vi "Create Analog DataSet MultiRow DataQ.vi"(8 "error in (no error)":errorcluster, 9 "Select":T1, 10 "TaskName":string, 11 "DataQueues in":refnum<class "DataQueues.lvclass">) -> (0 "error out":errorcluster, 2 "TaskName out":string, 3 "DataQueues out":refnum<class "DataQueues.lvclass">)   [LabVIEW 2017, in "DataQueues.lvclass"]
doc: "Developed by Kevin Thompson\nkevin@thompsonengineering.net\n\nCopyright 2018-2020\nThompson Engineering, LLC"
uses:
  DataQueues.lvclass
  DataTypes/DataQ SelectType--enum.ctl
  DataTypes/Analog DataSet MultiRow--cluster.ctl
  DataTypes/DataQ Ref DictNode--cluster.ctl
  DataQueues.lvclass/DataQueues.ctl
  Accessors/Get QueueNames.vi
  Accessors/Get DataQ Dict.vi
  Accessors/Set QueueNames.vi
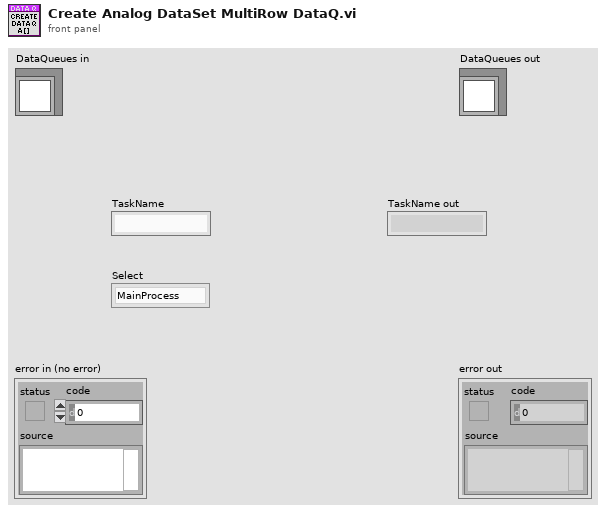
[diagram p1: front panel]
types:
  T1 = typedef "DataQueues.lvclass/DataQ SelectType--enum.ctl" = enum16{"MainProcess", "LogEngine", "LocalDAQThread"}
  T2 = typedef "DataQueues.lvclass/DataQ Ref DictNode--cluster.ctl" = cluster{"KeyName":string, "Type Name":string, "vDataQ Ref":variant}
  T3 = typedef "DataQueues.lvclass/Analog DataSet MultiRow--cluster.ctl" = cluster{"TimeStamp_(s)":dbl, "data":dbl[][]}
  T4 = typedef "TD Dynamic CVT DVR--ref.ctl" = refnum<data-value>
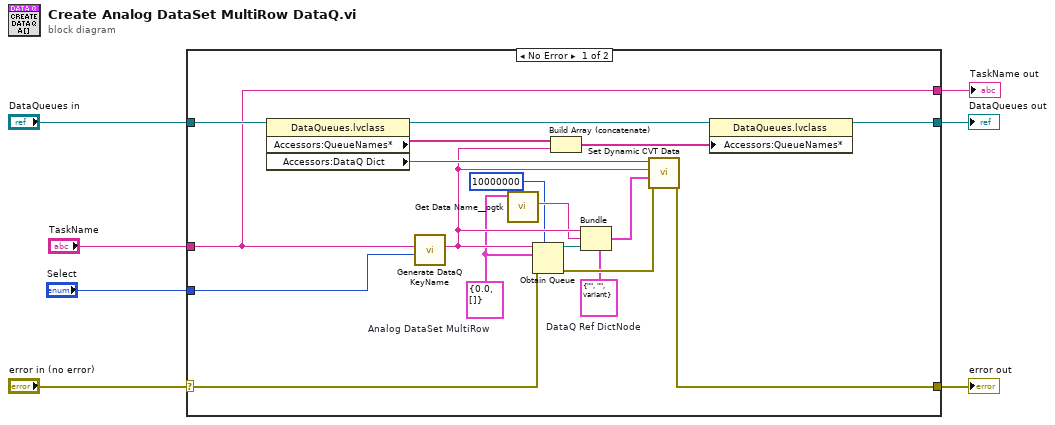
[diagram p0: block diagram]
diagram:
  n1 = case shown="No Error" "error in (no error)" {
    selector: "error in (no error)" -> [w23 w28]
    tunnel: [w22 w28] -> w6
    tunnel: [w21 w27] -> w4
    tunnel: "DataQueues in" -> [w19 w27]
    tunnel: "TaskName" -> [w9 w26]
    tunnel: "Select" -> [w25 _]
    tunnel: [w9 w26] -> w1
    frame No Error {
      w10 = T2 {"KeyName"="", "Type Name"="", "vDataQ Ref"=variant(refnum<queue> refnum)}  # DataQ Ref DictNode
      w11 = T3 {"TimeStamp_(s)"=0.0, "data"=[]}  # Analog DataSet MultiRow
      n2 = property class="DataQueues.lvclass"(reference=w19) -> (reference out=w18:refnum<class "DataQueues.lvclass">, "Accessors:QueueNames*"=w17:string[], "Accessors:DataQ Dict"=w20:T4)  [unwired: 1 in, 1 out]
      n3 = call "Generate DataQ KeyName.vi"("Select"=w25, "TaskName"=w9) -> ("DataQ KeyName"=w14:string)  [unwired: 9 in]
      n4 = call <userlib>:"Get Data Name__ogtk.vi"("Data"=w11) -> ("Data Name"=w12:string)  [unwired: 8 in, 2 out]
      n5 = Obtain Queue(max queue size (-1, unlimited)=10000000, name (unnamed)=w14, element data type=w11, error in (no error)=w23) -> (queue out=w15:refnum<queue>, error out=w24:errorcluster)  [unwired: 1 in, 1 out]
      n6 = Build Array (concatenate)(w17, w14) -> (w16:string[])
      n7 = Bundle(cluster=w10, "KeyName"=w14, "Type Name"=w12, "vDataQ Ref"=w15) -> (w13:T2)
      n8 = call <vilib>:"Set Dynamic CVT Data.vi"("error in (no error)"=w24, "value"=w13, "DataName"=w14, "dCVT DVR"=w20) -> ("error out"=w22:errorcluster)  [unwired: 5 in, 2 out]
      n9 = property class="DataQueues.lvclass"(reference=w18, "Accessors:QueueNames*"=w16) -> (reference out=w21:refnum<class "DataQueues.lvclass">)  [unwired: 1 in, 1 out]
    }
    frame Error {
    }
  }
  "error out" <- w6
  "DataQueues out" <- w4
  "TaskName out" <- w1
